vi "Cauchy Inverse CDF.vi"(9 "b":dbl=1.0, 10 "a":dbl=1.0, 11 "cdf(x)":dbl=0.4) -> (0 "error":i32, 3 "x":dbl=0.6750803037670938)   [LabVIEW 2020, in "NI_Gmath.lvlib"]
doc: "Computes the continuous inverse cumulative distribution function (CDF) of the various distributions. You must manually select the polymorphic instance to use."
uses:
  <vilib>/gmath/NI_Gmath.lvlib
  <vilib>/gmath/statdist.llb/st_error_code.ctl
panel:
  # "Cauchy Inverse CDF"
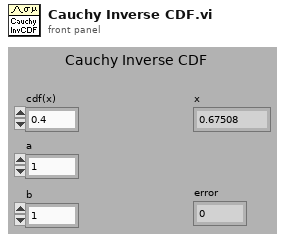
[diagram p1: front panel]
types:
  T1 = typedef "NI_Gmath.lvlib/st_error_code.ctl" = i32
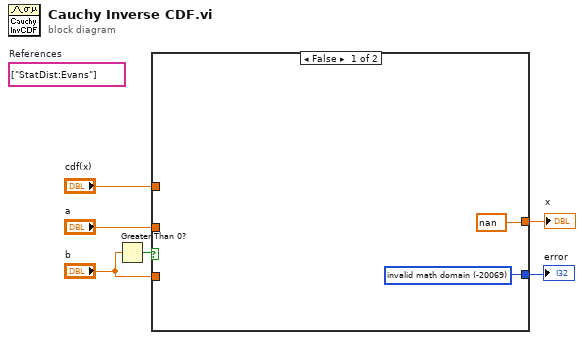
[diagram p0: block diagram]
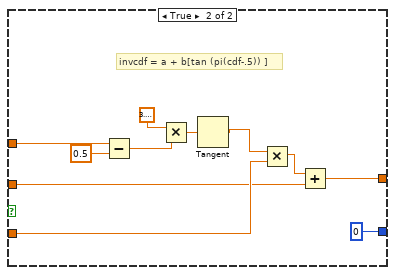
[diagram p2: hidden frame]
diagram:
  (unwired) string[] ["StatDist:Evans"]  # References
  n1 = Greater Than 0?(x="b") -> (x > 0?=w6:bool)
  n2 = case shown="False" w6 {
    tunnel: "b" -> [_ w12]
    tunnel: [w7 0 ("invalid math domain")] -> w4
    tunnel: [nan w9] -> w3
    tunnel: "cdf(x)" -> [_ w15]
    tunnel: "a" -> [_ w10]
    frame False {
      w7 = T1 -20069 items=["invalid math domain"=-20069, "Fourier interpolation size m >= n"=-20070, "empty array"=-20003] ("stat interp error code")
    }
    frame True {
      # "invcdf = a + b[tan (pi(cdf-.5)) ]"
      n3 = Subtract(x=w15, y=0.5) -> (x-y=w18:dbl)
      n4 = Multiply(x=3.141592653589793, y=w18) -> (x*y=w14:dbl)
      n5 = Tangent(1:w14) -> (0:w13:dbl)
      n6 = Multiply(x=w13, y=w12) -> (x*y=w11:dbl)
      n7 = Add(x=w11, y=w10) -> (x+y=w9:dbl)
    }
  }
  "x" <- w3
  "error" <- w4
